vi "continuously_read_current.vi"() -> ()   [LabVIEW 2024]
doc: "Configures a sweep and takes voltage and current readings at each point."
uses:
  Keithley 2450.lvlib
panel:
  in  "Limit Reached 2":bool
  in  "VISA resource name 2":refnum<visa-resource-name>="GPIB0::24::INSTR"
  in  "error in (no error)":errorcluster
  out "error out":errorcluster
  out "Current":dbl caption="Measured Current (A)"
  in  "stop":bool
  out "XY Graph":cluster{dbl[], dbl[]}(graph)
  in  "Measure Interval (ms)":u32
  in  "Max Elapsed time (s)":u32
  in  "Voltage Output Level (0)":dbl
  in  "Current Compliance Limit (0.1)":dbl=0.1
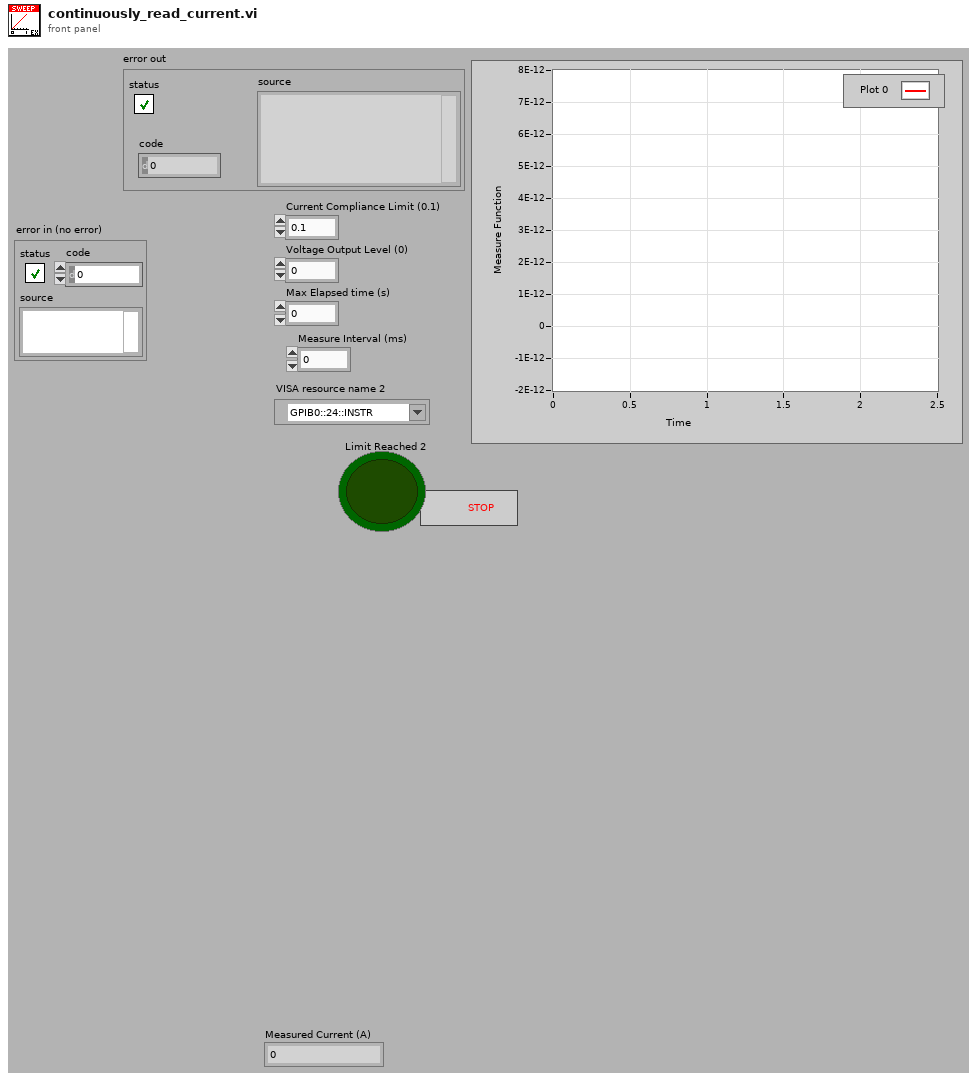
[diagram p1: front panel]
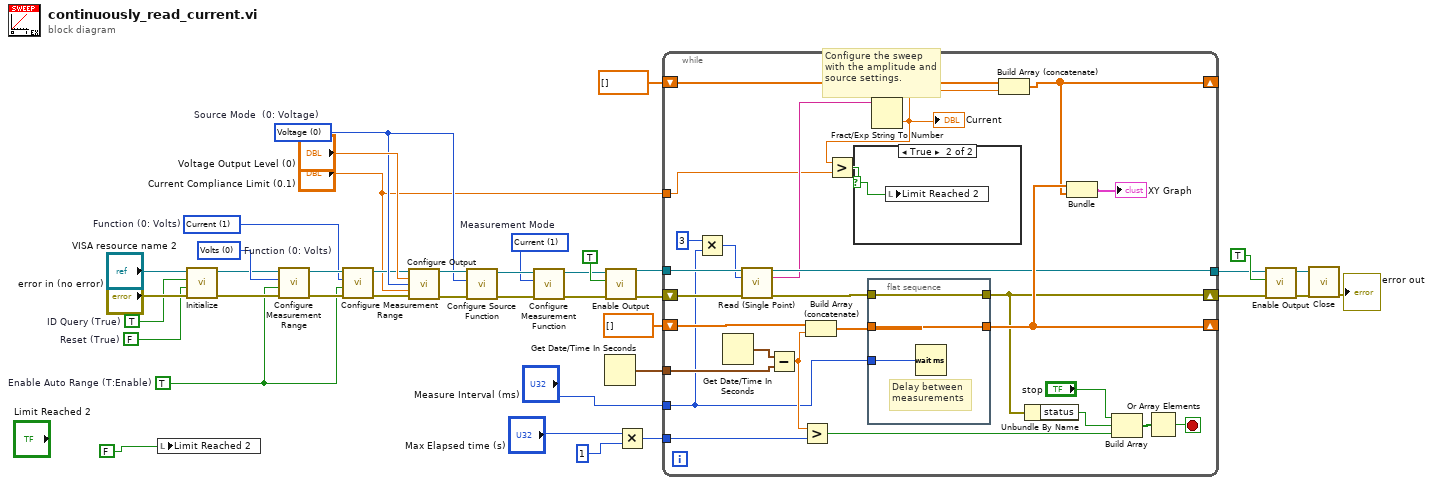
[diagram p0: block diagram]
diagram:
  w24 = u16 0 items=["Voltage", "Current"]  # Source Mode  (0: Voltage)
  w4 = u16 1 items=["Volts", "Current", "Auto Resistance", "Manual Resistance", "Digitize Voltage", "Digitize Current"]  # Measurement Mode
  w20 = TRUE  # Enable Auto Range (T:Enable)
  w30 = u16 1 items=["Volts", "Current", "Resistance"]  # Function (0: Volts)
  w31 = u16 0 items=["Volts", "Current", "Resistance"]  # Function (0: Volts)
  w22 = FALSE  # Reset (True)
  w21 = TRUE  # ID Query (True)
  # "Configure the sweep with the amplitude and source settings."
  n1 = local write "Limit Reached 2"(FALSE) -> ()
  n2 = call "Initialize.vi"("error in (no error)"="error in (no error)", "Reset (True)"=w22, "ID Query (True)"=w21, "VISA resource name"="VISA resource name 2") -> ("error out"=w27:errorcluster, "VISA resource name out"=w28:refnum<visa-resource-name>)  [unwired: 6 in]
  n3 = call "Configure Measurement Range.vi"("error in (no error)"=w27, "Enable Auto Range (T:Enable)"=w20, "Function (0: Volts)"=w31, "VISA resource name"=w28) -> ("error out"=w32:errorcluster, "VISA resource name out"=w33:refnum<visa-resource-name>)  [unwired: 6 in]
  n4 = call "Configure Measurement Range.vi"("error in (no error)"=w32, "Enable Auto Range (T:Enable)"=w20, "Function (0: Volts)"=w30, "VISA resource name"=w33) -> ("error out"=w6:errorcluster, "VISA resource name out"=w5:refnum<visa-resource-name>)  [unwired: 6 in]
  n5 = call "Configure Output.vi"("VISA resource name"=w5, "Source Level (0)"="Voltage Output Level (0)", "Source Mode  (0: Voltage)"=w24, "Source Limit Level (0.1)"="Current Compliance Limit (0.1)", "error in (no error)"=w6) -> ("VISA resource name out"=w26:refnum<visa-resource-name>, "error out"=w25:errorcluster)  [unwired: 9 in]
  n6 = call "Configure Source Function.vi"("error in (no error)"=w25, "Function (0: Volts)"=w24, "VISA resource name"=w26) -> ("error out"=w19:errorcluster, "VISA resource name out"=w18:refnum<visa-resource-name>)  [unwired: 7 in]
  n7 = call "Configure Measurement Function.vi"("error in (no error)"=w19, "Function (0: Volts)"=w4, "VISA resource name"=w18) -> ("error out"=w15:errorcluster, "VISA resource name out"=w14:refnum<visa-resource-name>)  [unwired: 7 in]
  n8 = Get Date/Time In Seconds() -> (seconds since 1Jan1904=w40:timestamp)
  n9 = call "Enable Output.vi"("error in (no error)"=w15, "Enable Output (T: Enable)"=TRUE, "VISA resource name"=w14) -> ("error out"=w16:errorcluster, "VISA resource name out"=w7:refnum<visa-resource-name>)  [unwired: 7 in]
  n10 = Multiply(x="Max Elapsed time (s)", y=u32 1) -> (x*y=w34:u32)
  n11 = while {
    shift-right: [w49] -> w10
    shift-left: w16 -> [w52]
    tunnel: w40 -> [w66]
    shift-right: [w60] -> _
    shift-left: dbl[] [] -> [w65]
    shift-right: [w59] -> _
    shift-left: dbl[] [] -> [w64]
    tunnel: "Measure Interval (ms)" -> [w47]
    tunnel: w34 -> [w56]
    tunnel: [w45] -> w9
    tunnel: w7 -> [w50]
    tunnel: "Current Compliance Limit (0.1)" -> [w42]
    stop <- w63 stop-if-true
    n12 = Multiply(x=u32 3, y=w47) -> (x*y=w48:u32)
    n13 = Get Date/Time In Seconds() -> (seconds since 1Jan1904=w67:timestamp)
    n14 = call "Read (Single Point).vi"("VISA resource name"=w50, "Timeout (10000 ms)"=w48, "error in (no error)"=w52) -> ("VISA resource name out"=w45:refnum<visa-resource-name>, "Data out"=w44:string, "error out"=w51:errorcluster)  [unwired: 10 in]
    n15 = Subtract(x=w67, y=w66) -> (x-y=w57:dbl)
    n16 = Greater?(x=w57, y=w56) -> (0:w53:bool)
    n17 = Build Array (concatenate)(w65, w57) -> (w61:dbl[])
    n18 = flat-sequence {
      tunnel: w61 -> [w71]
      tunnel: [w71] -> w60
      tunnel: w47 -> [w70]
      tunnel: w51 -> [w69]
      tunnel: [w69] -> w49
      frame #0 {
        # "Delay between\nmeasurements"
        n19 = Wait (ms)(milliseconds to wait=w70) -> ()  [unwired: 1 out]
      }
    }
    n20 = Fract/Exp String To Number(string=w44) -> (number=w43:dbl)  [unwired: 3 in, 1 out]
    "Current" <- w43
    n21 = Greater?(x=w43, y=w42) -> (0:w41:bool)
    n22 = case shown="True" w41 {
      selector: w41 -> [_ w68]
      frame False {
      }
      frame True {
        n23 = local write "Limit Reached 2"(w68) -> ()
      }
    }
    n24 = Build Array (concatenate)(w64, w43) -> (w59:dbl[])
    n25 = Unbundle By Name(w49) -> ("status"=w54:bool)
    n26 = Bundle(w60, w59) -> (→"XY Graph":cluster{dbl[], dbl[]})  [unwired: 1 in]
    n27 = Build Array("stop", w54, w53) -> (w62:bool[])
    n28 = Or Array Elements(Boolean array=w62) -> (logical OR=w63:bool)
  }
  n29 = call "Enable Output.vi"("error in (no error)"=w10, "Enable Output (T: Enable)"=TRUE, "VISA resource name"=w9) -> ("error out"=w11:errorcluster, "VISA resource name out"=w12:refnum<visa-resource-name>)  [unwired: 7 in]
  n30 = call "Close.vi"("error in (no error)"=w11, "VISA resource name"=w12) -> ("error out"=→"error out":errorcluster)  [unwired: 9 in]
